vi "create.TradeShort.vi"(8 "error in":errorcluster, 10 "TradeShort.Parameters":T1={"Time Offset"=447000, "Order Id"="ORID0001", "Execution Id"="EXE_ID_1", "Quantity"=20000, "Price"=0.905, "Side Indicator"="B", "Symbol"="AAPL"}, 11 "TradeShort in":refnum<class "TradeShort.lvclass">) -> (0 "error out":errorcluster, 3 "TradeShort out":refnum<class "TradeShort.lvclass">)   [LabVIEW 2020, in "TradeShort.lvclass"]
uses:
  TradeShort.lvclass
  TradeShort.Parameters.ctl
  FieldSpec.ctl
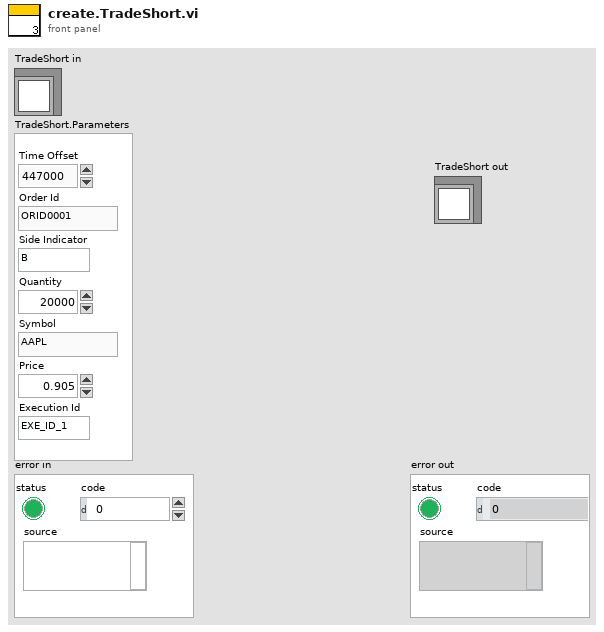
[diagram p1: front panel]
types:
  T1 = typedef "TradeShort.lvclass/TradeShort.Parameters.ctl" = cluster{"Time Offset":u32, "Order Id":string, "Execution Id":string, "Quantity":u32, "Price":dbl, "Side Indicator":string, "Symbol":string}
  T2 = typedef "FieldSpec.ctl" = cluster{"Name":string, "Offset":i32, "Length":i32, "FieldType":enum16{"Alphanumeric", "Binary", "BinaryLongPrice", "BinaryShortPrice", "BitField", "PrintableAscii", "Value"}, "FieldValue":variant}
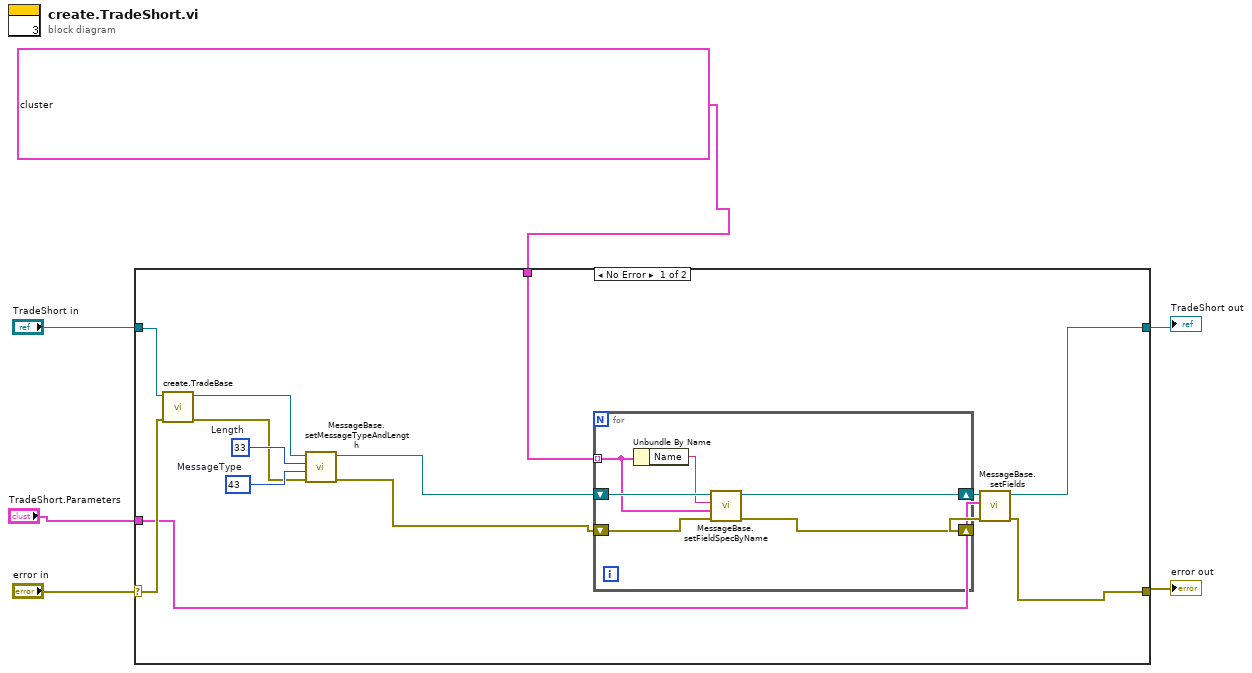
[diagram p0: block diagram]
diagram:
  n1 = case shown="No Error" "error in" {
    selector: "error in" -> [w15 w28]
    tunnel: [w10 w28] -> w5
    tunnel: [w12 w27] -> w3
    tunnel: "TradeShort in" -> [w16 w27]
    tunnel: T2[] [{"Name"="Quantity", "Offset"=15, "Length"=2, "FieldType"=enum."Binary", "FieldValue"=variant}, {"Name"="Symbol", "Offset"=17, "Length"=6, "FieldType"=enum."PrintableAscii", "FieldValue"=variant}, {"Name"="Price", "Offset"=23, "Length"=2, "FieldType"=enum."BinaryShortPrice", "FieldValue"=variant}, {"Name"="Execution Id", "Offset"=25, "Length"=8, "FieldType"=enum."PrintableAscii", "FieldValue"=variant}] ("appended array") -> [w8 _]
    tunnel: "TradeShort.Parameters" -> [w7 _]
    frame No Error {
      w19 = u8 43  # MessageType
      w20 = u8 33  # Length
      n2 = call-dynamic "create.TradeBase.vi"("error in (no error)"=w15, "TradeBase in"=w16) -> ("error out"=w18:errorcluster, "TradeBase out"=w17:refnum<class "TradeShort.lvclass">)  [unwired: 8 in]
      n3 = call-dynamic "MessageBase.setMessageTypeAndLength.vi"("error in (no error)"=w18, "MessageType"=w19, "Length"=w20, "MessageBase in"=w17) -> ("error out"=w9:errorcluster, "MessageBase out"=w11:refnum<class "TradeShort.lvclass">)  [unwired: 6 in]
      n4 = for {
        tunnel: w8 -> [w23] mode=indexing
        shift-right: [w22] -> w14
        shift-left: w11 -> [w26]
        shift-right: [w21] -> w13
        shift-left: w9 -> [w25]
        n5 = Unbundle By Name(w23) -> ("Name"=w24:string)
        n6 = call-dynamic "MessageBase.setFieldSpecByName.vi"("error in (no error)"=w25, "FIeldSpec"=w23, "Field.Name"=w24, "MessageBase in"=w26) -> ("error out"=w21:errorcluster, "MessageBase out"=w22:refnum<class "TradeShort.lvclass">)  [unwired: 6 in]
      }
      n7 = call-dynamic "MessageBase.setFields.vi"("error in (no error)"=w13, "Cluster (dup)"=w7, "MessageBase in"=w14) -> ("error out"=w10:errorcluster, "MessageBase out"=w12:refnum<class "TradeShort.lvclass">)  [unwired: 7 in]
    }
    frame Error {
    }
  }
  "error out" <- w5
  "TradeShort out" <- w3
